vi "BasicUIExample.vi"() -> ()   [LabVIEW 2020]
uses:
  PalmSens/PalmSens.lvclass
  D:/PalmSensAppsAndSDKS/LabVIEW/PalmSens SDK for LabVIEW 5.10/PalmSens/Libraries/PalmSens.Core.dll
  PalmSens/Libraries/PalmSens.Core.dll
  PalmSens/LiveCurveResult.ctl
panel:
  out "Curve Value Count":i32
  out "Live Curve Result":T1
  out "Stopped":bool
  out "Is Measuring":bool
  out "Abort Measurement":bool
  out "Method .NET":refnum<k24>
  out "XY Graph":cluster{"X":dbl, "Y":dbl}[](graph)
  in  "Abort button":bool
  in  "Measure button":bool
  in  "Disconnect Button":bool
  in  "Connect Button":bool
  out "PalmSens.lvclass":refnum<class "PalmSens.lvclass">
  in  "stop":bool
  in  "Scan Button":bool
  in  "Available Instruments":i32(listbox)
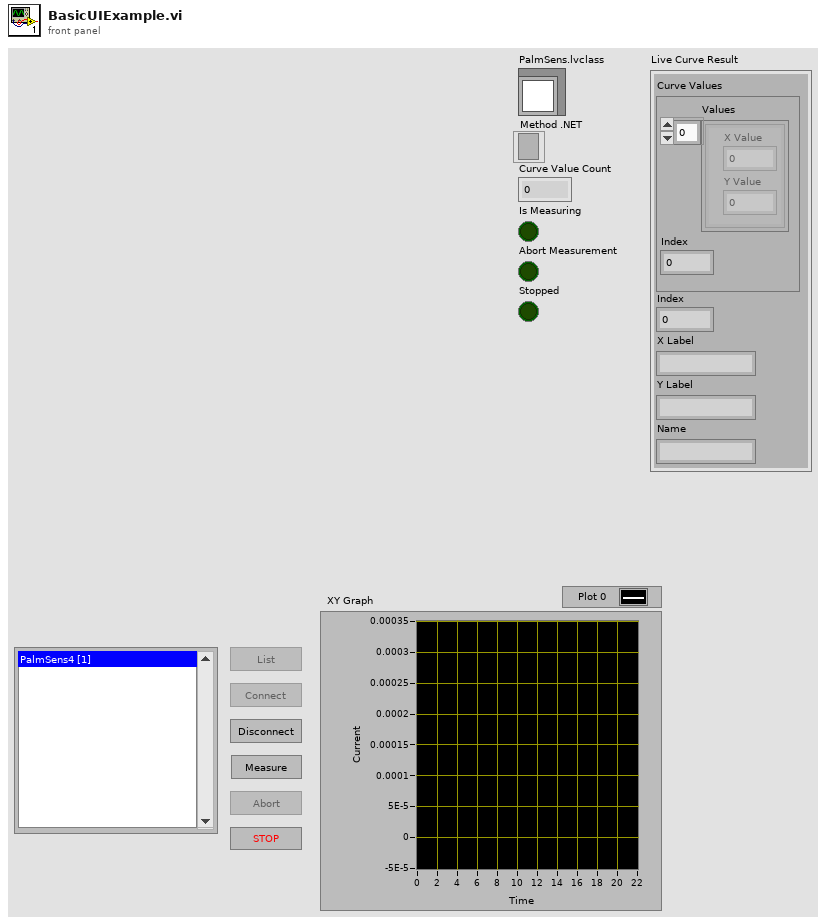
[diagram p1: front panel]
types:
  T1 = typedef "LiveCurveResult.ctl" = cluster{"X Label":string, "Y Label":string, "Name":string, "Index":i16, "Curve Values":cluster{"Values":cluster{"X Value":dbl, "Y Value":dbl}[], "Index":i16}}
  T2 = enum8{"Enabled", "Disabled", "Disabled and Grayed Out"}
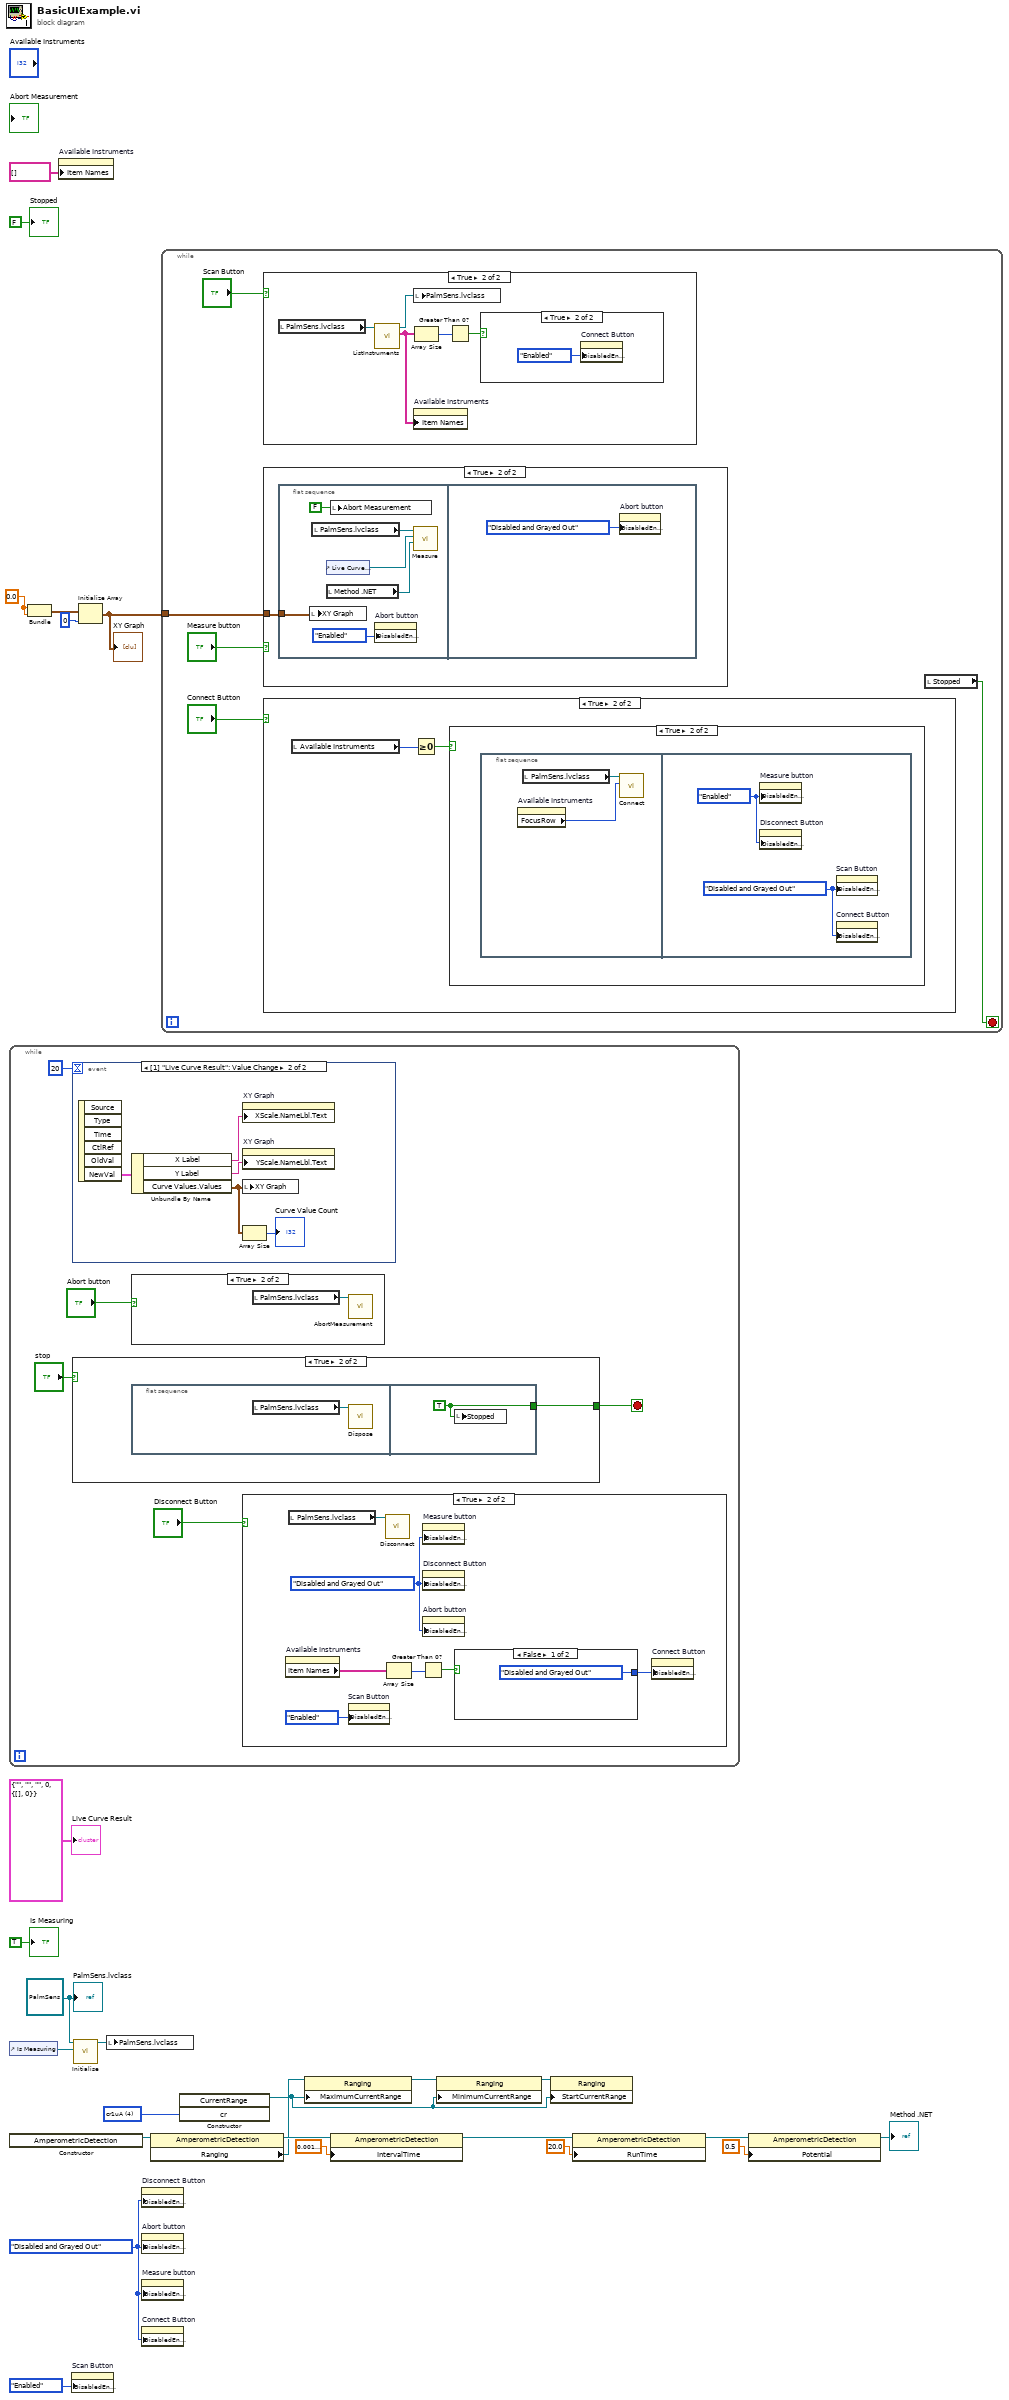
[diagram p0: block diagram]
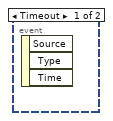
[diagram p2: hidden frame]
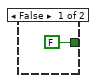
[diagram p3: hidden frame]
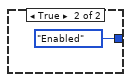
[diagram p6: hidden frame]
diagram:
  w5 = 4 items=["cr100pA"=0, "cr1nA"=1, "cr10nA"=2, "cr100nA"=3, "cr1uA"=4, "cr10uA"=5, "cr100uA"=6, "cr1mA"=7, "cr10mA"=8, "cr100mA"=9, "cr2uA"=10, "cr4uA"=11, "cr8uA"=12, "cr16uA"=13, "cr32uA"=14, "cr125uA"=17, "cr250uA"=18, "cr500uA"=19, "cr5mA"=20, "cr6uA"=21, "cr13uA"=22, "cr25uA"=23, "cr50uA"=24, "cr200uA"=25, "cr63uA"=26] ("cr")
  w16 = 0.0
  w17 = T2."Disabled and Grayed Out" ("Disabled")
  w26 = refnum<class "PalmSens.lvclass"> refnum ("PalmSens.lvclass")
  n1 = while {
    stop <- w28 stop-if-true
    n2 = event shown="[1] \"Live Curve Result\": Value Change" {
      selector: _ -> [_ _]
      dyn-events: _ -> [_ _]
      timeout: 20 -> [_ _]
      event Timeout {
        n3 = event-data() -> ()  [unwired: 1 in, 3 out]
      }
      event Value Change {
        n4 = event-data() -> ("NewVal"=w36:T1)  [unwired: 1 in, 5 out]
        n5 = Unbundle By Name(w36) -> ("X Label"=w34:string, "Y Label"=w35:string, "Curve Values.Values"=w33:cluster{"X Value":dbl, "Y Value":dbl}[])
        n6 = local write "XY Graph"(w33) -> ()
        n7 = Array Size(array=w33) -> (size(s)=→"Curve Value Count":i32)
        n8 = property on="XY Graph" class="XYGraph (strict)"("XScale.NameLbl.Text"=w34) -> ()  [unwired: 2 in, 2 out]
        n9 = property on="XY Graph" class="XYGraph (strict)"("YScale.NameLbl.Text"=w35) -> ()  [unwired: 2 in, 2 out]
      }
    }
    n10 = case shown="True" "stop" {
      tunnel: [FALSE w38] -> w28
      frame False {
      }
      frame True {
        n11 = flat-sequence {
          tunnel: [w40] -> w38
          frame #0 {
            n12 = local read "PalmSens.lvclass"() -> (w39:refnum<class "PalmSens.lvclass">)
            n13 = call-dynamic "Dispose.vi"("PalmSens in"=w39) -> ()  [unwired: 9 in, 2 out]
          }
          frame #1 {
            w40 = TRUE
            n14 = local write "Stopped"(w40) -> ()
          }
        }
      }
    }
    n15 = case shown="True" "Abort button" {
      frame False {
      }
      frame True {
        n16 = local read "PalmSens.lvclass"() -> (w41:refnum<class "PalmSens.lvclass">)
        n17 = call-dynamic "AbortMeasurement.vi"("PalmSens in"=w41) -> ()  [unwired: 9 in, 2 out]
      }
    }
    n18 = case shown="True" "Disconnect Button" {
      frame False {
      }
      frame True {
        w47 = T2."Disabled and Grayed Out" ("Disabled")
        n19 = property on="Available Instruments" class="LstBox (strict)"() -> ("Item Names"=w46:string[])  [unwired: 2 in, 2 out]
        n20 = local read "PalmSens.lvclass"() -> (w42:refnum<class "PalmSens.lvclass">)
        n21 = property on="Scan Button" class="Bool"("DisabledEnum"=T2."Enabled" ("Disabled")) -> ()  [unwired: 2 in, 2 out]
        n22 = call-dynamic "Disconnect.vi"("PalmSens in"=w42) -> ()  [unwired: 9 in, 2 out]
        n23 = Array Size(array=w46) -> (size(s)=w45:i32)
        n24 = Greater Than 0?(x=w45) -> (x > 0?=w44:bool)
        n25 = property on="Measure button" class="Bool"("DisabledEnum"=w47) -> ()  [unwired: 2 in, 2 out]
        n26 = property on="Disconnect Button" class="Bool"("DisabledEnum"=w47) -> ()  [unwired: 2 in, 2 out]
        n27 = property on="Abort button" class="Bool"("DisabledEnum"=w47) -> ()  [unwired: 2 in, 2 out]
        n28 = case shown="False" w44 {
          tunnel: [T2."Disabled and Grayed Out" ("Disabled") T2."Enabled" ("Disabled")] -> w43
          frame False {
          }
          frame True {
          }
        }
        n29 = property on="Connect Button" class="Bool"("DisabledEnum"=w43) -> ()  [unwired: 2 in, 2 out]
      }
    }
  }
  n30 = control-ref of="Is Measuring"() -> (w11:refnum<vi>)
  n31 = constructor class="AmperometricDetection"() -> (reference out=w8:refnum<k24>)  [unwired: 3 in, 2 out]
  n32 = Bundle(w16, w16) -> (w15:cluster{dbl, dbl})  [unwired: 1 in]
  n33 = property on="Available Instruments" class="LstBox (strict)"("Item Names"=string[] []) -> ()  [unwired: 2 in, 2 out]
  n34 = property on="Scan Button" class="Bool"("DisabledEnum"=T2."Enabled" ("Disabled")) -> ()  [unwired: 2 in, 2 out]
  n35 = call-dynamic "Initialise.vi"("Is Measuring Refnum"=w11, "PalmSens in"=w26) -> ("PalmSens out"=w25:refnum<class "PalmSens.lvclass">)  [unwired: 8 in, 1 out]
  n36 = Initialize Array(w15, 0 ("dimension size")) -> (w1:cluster{dbl, dbl}[])
  "XY Graph" <- w1
  n37 = local write "PalmSens.lvclass"(w25) -> ()
  n38 = property on="Disconnect Button" class="Bool"("DisabledEnum"=w17) -> ()  [unwired: 2 in, 2 out]
  n39 = property on="Abort button" class="Bool"("DisabledEnum"=w17) -> ()  [unwired: 2 in, 2 out]
  n40 = property on="Measure button" class="Bool"("DisabledEnum"=w17) -> ()  [unwired: 2 in, 2 out]
  n41 = property on="Connect Button" class="Bool"("DisabledEnum"=w17) -> ()  [unwired: 2 in, 2 out]
  n42 = property class="AmperometricDetection"(reference=w8) -> (reference out=w7:refnum<k24>, "Ranging"=w6:refnum<k24>)  [unwired: 1 in, 1 out]
  n43 = while {
    tunnel: w1 -> [w51]
    stop <- w52 stop-if-true
    n44 = case shown="True" "Scan Button" {
      frame False {
      }
      frame True {
        n45 = local read "PalmSens.lvclass"() -> (w74:refnum<class "PalmSens.lvclass">)
        n46 = call-dynamic "ListInstruments.vi"("PalmSens in"=w74) -> ("Array"=w72:string[], "PalmSens out"=w73:refnum<class "PalmSens.lvclass">)  [unwired: 8 in, 1 out]
        n47 = local write "PalmSens.lvclass"(w73) -> ()
        n48 = property on="Available Instruments" class="LstBox (strict)"("Item Names"=w72) -> ()  [unwired: 2 in, 2 out]
        n49 = Array Size(array=w72) -> (size(s)=w71:i32)
        n50 = Greater Than 0?(x=w71) -> (x > 0?=w70:bool)
        n51 = case shown="True" w70 {
          frame False {
          }
          frame True {
            n52 = property on="Connect Button" class="Bool"("DisabledEnum"=T2."Enabled" ("Disabled")) -> ()  [unwired: 2 in, 2 out]
          }
        }
      }
    }
    n53 = case shown="True" "Measure button" {
      tunnel: w51 -> [_ w56]
      frame False {
      }
      frame True {
        n54 = flat-sequence {
          tunnel: w56 -> [w61]
          frame #0 {
            n55 = local write "XY Graph"(w61) -> ()
            n56 = local read "PalmSens.lvclass"() -> (w62:refnum<class "PalmSens.lvclass">)
            n57 = control-ref of="Live Curve Result"() -> (w57:refnum<vi>)
            n58 = local read "Method .NET"() -> (w58:refnum<k24>)
            n59 = local write "Abort Measurement"(FALSE ("Abort button")) -> ()
            n60 = property on="Abort button" class="Bool"("DisabledEnum"=T2."Enabled" ("Disabled")) -> ()  [unwired: 2 in, 2 out]
            n61 = call-dynamic "Measure.vi"("Method .NET Refnum"=w58, "Live Curve Result Refnum"=w57, "PalmSens in"=w62) -> ()  [unwired: 1 in, 3 out]
          }
          frame #1 {
            n62 = property on="Abort button" class="Bool"("DisabledEnum"=T2."Disabled and Grayed Out" ("Disabled")) -> ()  [unwired: 2 in, 2 out]
          }
        }
      }
    }
    n63 = case shown="True" "Connect Button" {
      frame False {
      }
      frame True {
        n64 = local read "Available Instruments"() -> (w65:i32)
        n65 = Greater Or Equal To 0?(x=w65) -> (x >= 0?=w64:bool)
        n66 = case shown="True" w64 {
          frame False {
          }
          frame True {
            n67 = flat-sequence {
              frame #0 {
                n68 = property on="Available Instruments" class="LstBox (strict)"() -> ("FocusRow"=w66:i32)  [unwired: 2 in, 2 out]
                n69 = local read "PalmSens.lvclass"() -> (w67:refnum<class "PalmSens.lvclass">)
                n70 = call-dynamic "Connect.vi"("Instrument Index"=w66, "PalmSens in"=w67) -> ()  [unwired: 8 in, 2 out]
              }
              frame #1 {
                w69 = T2."Enabled" ("Disabled")
                w68 = T2."Disabled and Grayed Out" ("Disabled")
                n71 = property on="Measure button" class="Bool"("DisabledEnum"=w69) -> ()  [unwired: 2 in, 2 out]
                n72 = property on="Disconnect Button" class="Bool"("DisabledEnum"=w69) -> ()  [unwired: 2 in, 2 out]
                n73 = property on="Scan Button" class="Bool"("DisabledEnum"=w68) -> ()  [unwired: 2 in, 2 out]
                n74 = property on="Connect Button" class="Bool"("DisabledEnum"=w68) -> ()  [unwired: 2 in, 2 out]
              }
            }
          }
        }
      }
    }
    n75 = local read "Stopped"() -> (w52:bool)
  }
  n76 = constructor class="CurrentRange"("cr"=w5) -> (reference out=w2:refnum<k24>)  [unwired: 3 in, 3 out]
  n77 = property class="Ranging"(reference=w6, "MaximumCurrentRange"=w2) -> (reference out=w4:refnum<k24>)  [unwired: 1 in, 1 out]
  n78 = property class="AmperometricDetection"(reference=w7, "IntervalTime"=sgl 0.001) -> (reference out=w22:refnum<k24>)  [unwired: 1 in, 1 out]
  n79 = property class="Ranging"(reference=w4, "MinimumCurrentRange"=w2) -> (reference out=w3:refnum<k24>)  [unwired: 1 in, 1 out]
  n80 = property class="Ranging"(reference=w3, "StartCurrentRange"=w2) -> ()  [unwired: 1 in, 2 out]
  n81 = property class="AmperometricDetection"(reference=w22, "RunTime"=sgl 20.0) -> (reference out=w20:refnum<k24>)  [unwired: 1 in, 1 out]
  n82 = property class="AmperometricDetection"(reference=w20, "Potential"=sgl 0.5) -> (reference out=→"Method .NET":refnum<k24>)  [unwired: 1 in, 1 out]
  "PalmSens.lvclass" <- w26
  "Is Measuring" <- TRUE ("Is Measuring")
  "Stopped" <- FALSE ("Stopped")
  "Live Curve Result" <- T1 {"X Label"="", "Y Label"="", "Name"="", "Index"=0, "Curve Values"={"Values"=[], "Index"=0}} ("Live Curve Result")
